vi "signalReader.vi"(11 "Filename":path=path "G:/UCB/Instruments/tip making/Qplus AFM tip making/qplus test/Caihong/CJ39.xlsx") -> (1 "Step Size":dbl, 2 "Signal Column":i64[](array[numeric]), 3 "Frequency Column":i64[](array[numeric]))   [LabVIEW 2016]
uses:
  <vilib>/Utility/file.llb/Read Delimited Spreadsheet (I64).vi
panel:
  # "Reads a 2 column text file where the first column are the scanned frequencies\nand the second column is the signal response"
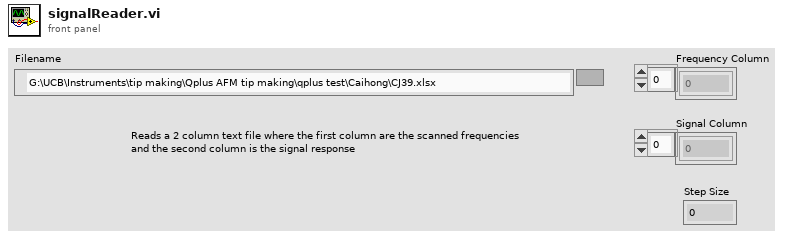
[diagram p1: front panel]
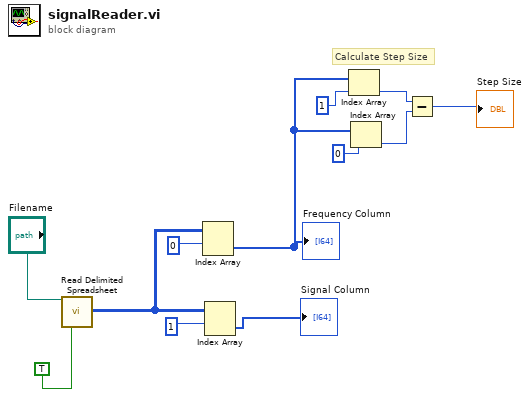
[diagram p0: block diagram]
diagram:
  # "Calculate Step Size"
  n1 = call-poly <vilib>:"Read Delimited Spreadsheet.vi"("file path (dialog if empty)"="Filename", "transpose? (F)"=TRUE) -> ("all rows"=w7:i64[][])  [unwired: 8 in, 5 out]
  n2 = Index Array(array=w7, index (row)=0) -> (element=w6:i64[])  [unwired: 1 in]
  "Frequency Column" <- w6
  n3 = Index Array(array=w7, index (row)=1) -> (element=→"Signal Column":i64[])  [unwired: 1 in]
  n4 = Index Array(array=w6, index=1) -> (element=w3:i64)
  n5 = Index Array(array=w6, index=0) -> (element=w2:i64)
  n6 = Subtract(x=w3, y=w2) -> (x-y=→"Step Size":i64)
